vi "Solenoid GetSet.vi"(9 "Enum":enum16{"Set", "Get", "Clear"}(ring), 10 "PneumaticsDevRef in":T1={"Pneumatic State Reference"=refnum, "SolenoidDevRef"={"DevStatus"={"status"=FALSE, "code"=0, "source"=""}, "Pneumatics Control Module"=0, "Forward Solenoid Channel"=enum."Invalid", "Reverse Solenoid Channel"=enum."Invalid"}, "Pneumatic Configuration reference"=refnum}, 11 "DevRef":string) -> (0 "Error Out":errorcluster, 3 "PneumaticsDevRef out":T1={"Pneumatic State Reference"=refnum, "SolenoidDevRef"={"DevStatus"={"status"=FALSE, "code"=0, "source"=""}, "Pneumatics Control Module"=0, "Forward Solenoid Channel"=enum."Invalid", "Reverse Solenoid Channel"=enum."Invalid"}, "Pneumatic Configuration reference"=refnum})   [LabVIEW 2015]
uses:
  <userlib>/836-Library/Pneumatics/Pneumatics/836_PneumaticsDevRef.ctl
  <userlib>/836-Library/Pneumatics/Pneumatics/Pneumatic State.ctl
  <userlib>/836-Library/Pneumatics/Pneumatics/StateMachine.ctl
  <vilib>/Rock Robotics/WPI/Solenoid/WPI_SolenoidDevRef.ctl
  <vilib>/Rock Robotics/WPI/Solenoid/WPI_SolenoidChannel.ctl
  <userlib>/836-Library/Pneumatics/Pneumatics/Pneumatic Configuration.ctl
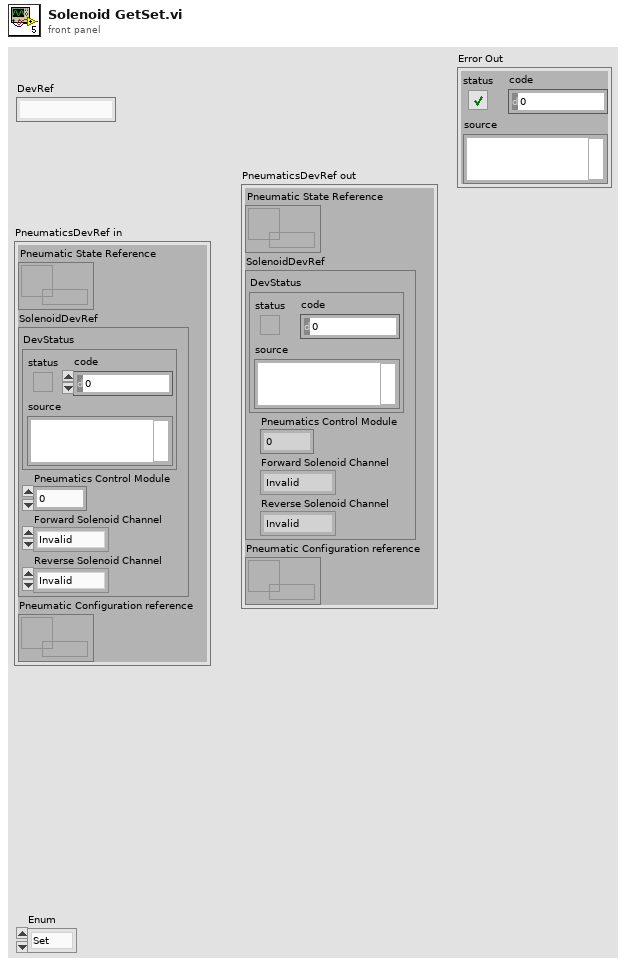
[diagram p1: front panel]
types:
  T1 = typedef "836_PneumaticsDevRef.ctl" = cluster{"Pneumatic State Reference":refnum<data-value>, "SolenoidDevRef":T2, "Pneumatic Configuration reference":refnum<data-value>}
  T2 = typedef "WPI_SolenoidDevRef.ctl" = cluster{"DevStatus":errorcluster, "Pneumatics Control Module":u8, "Forward Solenoid Channel":T3, "Reverse Solenoid Channel":T3}
  T3 = typedef "WPI_SolenoidChannel.ctl" = enum8{"Solenoid 0", "Solenoid 1", "Solenoid 2", "Solenoid 3", "Solenoid 4", "Solenoid 5", "Solenoid 6", "Solenoid 7", "Invalid"}
  T4 = typedef "Pneumatic State.ctl" = cluster{"Position":bool, "Initialize":bool, "Current State":T5, "Multiuse Timer A":u32, "Multiuse Timer B":u32}
  T5 = typedef "StateMachine.ctl" = enum8{"Status", "Forward", "Back", "Toggle", "Timed Forward", "Timed Back", "Analog Forwad", "Analog Back", "Digital Forward", "Digital Back", "Off", "Float", "Digital Forward Timeout", "Digital Back Timeout"}
  T6 = typedef "Pneumatic Configuration.ctl" = cluster{"Time Forward (ms)":u32, "Time Back (ms)":u32, "Digital Forward Time (ms)":u32, "Digital Backward Time (ms)":u32, "Analog Forward Settling Time (ms)":u32, "Analog Backward Settling Time (ms)":u32, "Analog Forward Threshold":sgl, "Analog Backward Threshold":sgl}
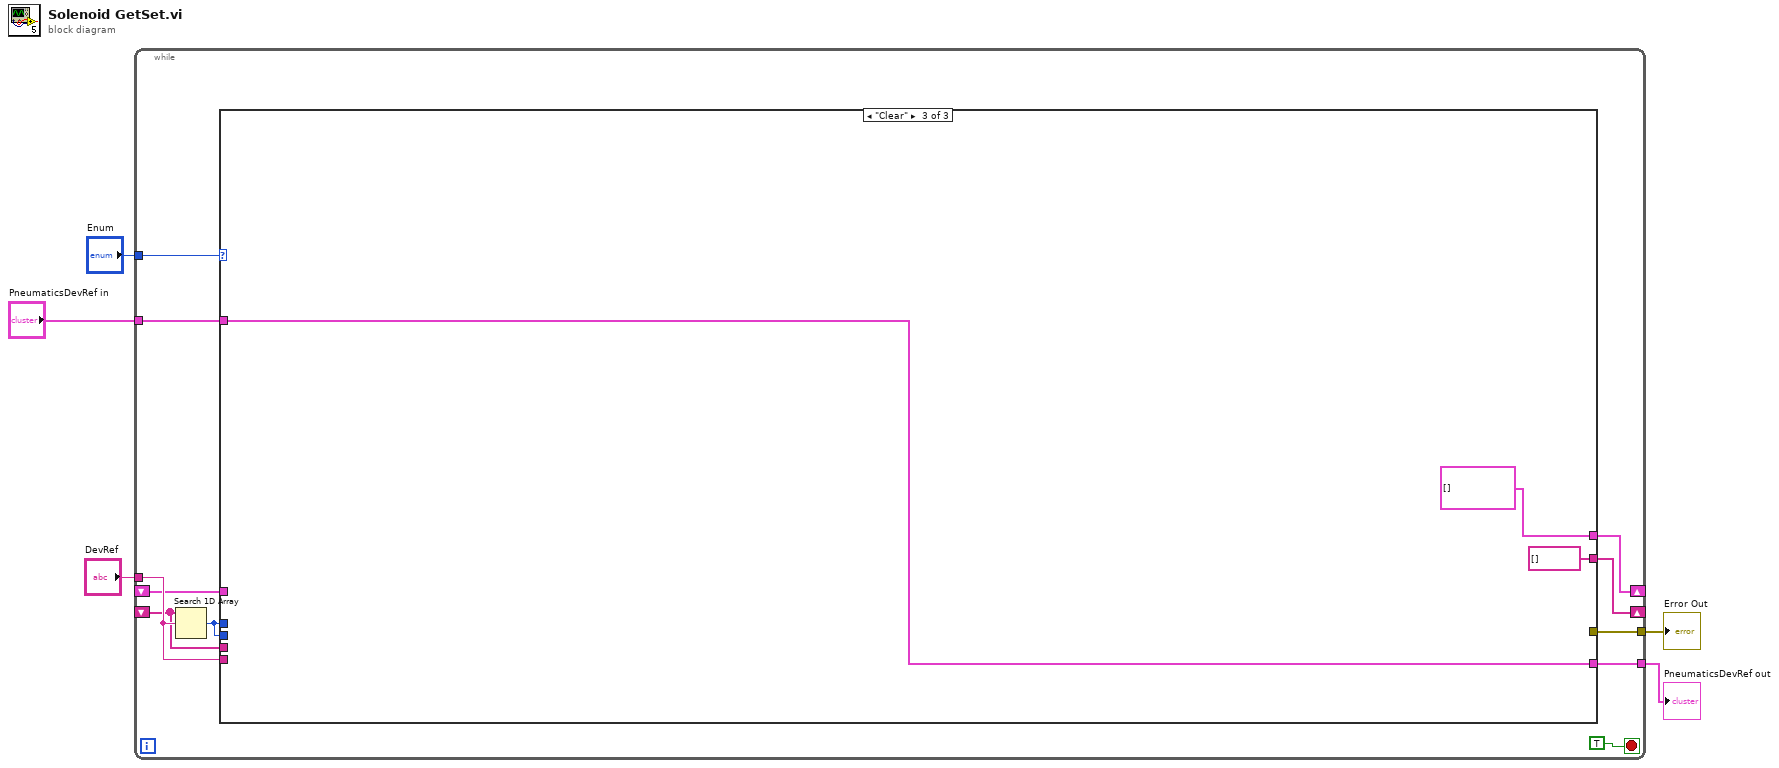
[diagram p0: block diagram]
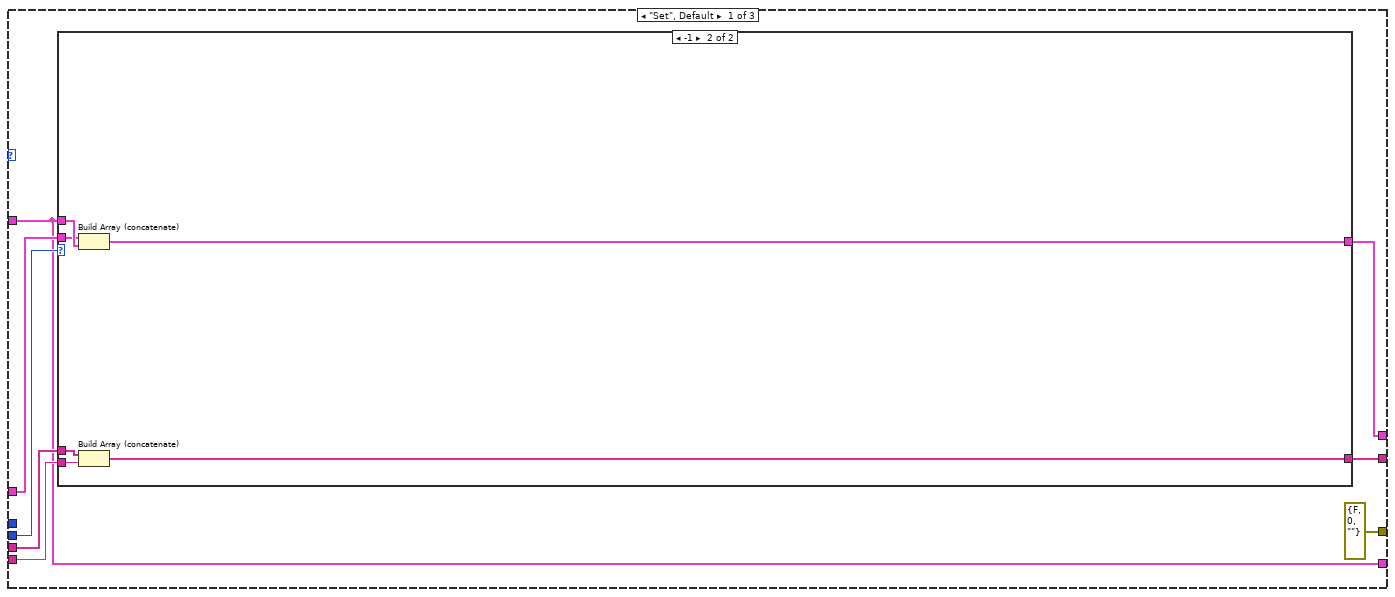
[diagram p2: hidden frame]
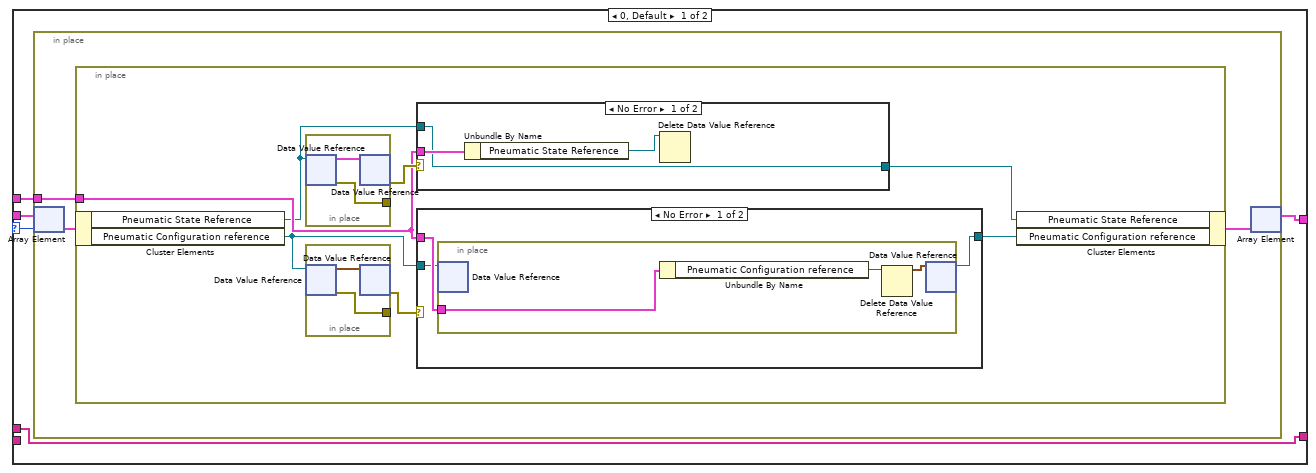
[diagram p3: hidden frame]
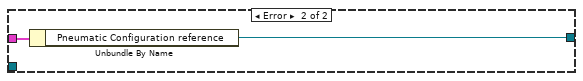
[diagram p4: hidden frame]
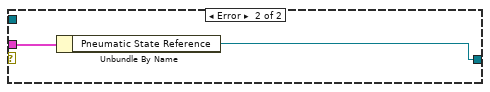
[diagram p5: hidden frame]
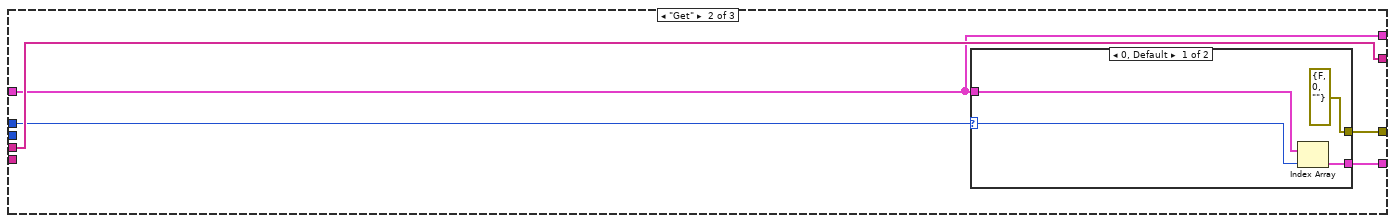
[diagram p6: hidden frame]
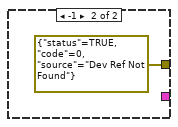
[diagram p7: hidden frame]
diagram:
  n1 = while {
    shift-right: [w12] -> _
    shift-left: _ -> [w11]
    shift-right: [w15] -> _
    shift-left: _ -> [w14]
    tunnel: "DevRef" -> [w16]
    tunnel: "PneumaticsDevRef in" -> [w13]
    tunnel: [w8] -> w4
    tunnel: "Enum" -> [w7]
    tunnel: [w6] -> w1
    stop <- TRUE stop-if-true
    n2 = Search 1D Array(1D array=w14, element=w16) -> (index of element=w9:i32)  [unwired: 1 out]
    n3 = case shown="\"Clear\"" w7 {
      tunnel: w9 -> [w24 _ _]
      tunnel: w16 -> [w23 _ _]
      tunnel: [w22 w67 string[] []] -> w15
      tunnel: w14 -> [w21 w67 _]
      tunnel: w13 -> [w18 _ w73]
      tunnel: [w20 w66 T1[] []] -> w12
      tunnel: w11 -> [w19 w66 _]
      tunnel: w9 -> [_ w65 _]
      tunnel: [w18 w64 w73] -> w8
      tunnel: [errorcluster {"status"=FALSE, "code"=0, "source"=""} ("error constant") w63 _] -> w6
      frame "Set", Default {
        n4 = case shown="-1" w24 {
          selector: w24 -> [w29 _]
          tunnel: [w25 w62] -> w20
          tunnel: [w28 w61] -> w22
          tunnel: w23 -> [_ w60]
          tunnel: w21 -> [w28 w59]
          tunnel: w18 -> [w26 w58]
          tunnel: w19 -> [w27 w57]
          frame 0, Default {
            n5 = in-place {
              in-place-border: w26 -> [w31]
              n6 = in-place-array #1(w27, w29) -> (w32:T1)
              n7 = in-place {
                in-place-border: w31 -> [w38]
                n8 = in-place-cluster #2(w32) -> ("Pneumatic State Reference"=w36:refnum<data-value>, "Pneumatic Configuration reference"=w35:refnum<data-value>)
                n9 = in-place {
                  in-place-border: [w56] -> _
                  n10 = in-place-dvr #3(w36) -> (w55:T4, w56:errorcluster)
                  n11 = in-place-dvr #3(w55) -> (w39:errorcluster)  [unwired: 1 out]
                }
                n12 = in-place {
                  in-place-border: [w54] -> _
                  n13 = in-place-dvr #4(w35) -> (w53:T6, w54:errorcluster)
                  n14 = in-place-dvr #4(w53) -> (w33:errorcluster)  [unwired: 1 out]
                }
                n15 = case shown="No Error" w39 {
                  tunnel: w38 -> [w50 w52]
                  tunnel: [w48 w51] -> w37
                  tunnel: w36 -> [w48 _]
                  frame No Error {
                    n16 = Unbundle By Name(w50) -> ("Pneumatic State Reference"=w49:refnum<data-value>)
                    n17 = Delete Data Value Reference(data value reference=w49) -> ()  [unwired: 1 in, 2 out]
                  }
                  frame Error {
                    n18 = Unbundle By Name(w52) -> ("Pneumatic State Reference"=w51:refnum<data-value>)
                  }
                }
                n19 = case shown="No Error" w33 {
                  tunnel: w38 -> [w42 w47]
                  tunnel: w35 -> [w41 _]
                  tunnel: [w40 w46] -> w34
                  frame No Error {
                    n20 = in-place {
                      in-place-border: w42 -> [w45]
                      n21 = in-place-dvr #5(w41) -> ()  [unwired: 2 out]
                      n22 = Unbundle By Name(w45) -> ("Pneumatic Configuration reference"=w44:refnum<data-value>)
                      n23 = Delete Data Value Reference(data value reference=w44) -> (data value=w43:T6)  [unwired: 1 in, 1 out]
                      n24 = in-place-dvr #5(w43) -> (w40:refnum<data-value>)  [unwired: 1 out]
                    }
                  }
                  frame Error {
                    n25 = Unbundle By Name(w47) -> ("Pneumatic Configuration reference"=w46:refnum<data-value>)
                  }
                }
                n26 = in-place-cluster #2("Pneumatic State Reference"=w37, "Pneumatic Configuration reference"=w34) -> (w30:T1)
              }
              n27 = in-place-array #1(w30) -> (w25:T1[])  [unwired: 1 out]
            }
          }
          frame -1 {
            n28 = Build Array (concatenate)(w57, w58) -> (w62:T1[])
            n29 = Build Array (concatenate)(w59, w60) -> (w61:string[])
          }
        }
      }
      frame "Get" {
        n30 = case shown="0, Default" w65 {
          selector: w65 -> [w70 _]
          tunnel: w66 -> [w71 _]
          tunnel: [w69 _] -> w64
          tunnel: [errorcluster {"status"=FALSE, "code"=0, "source"=""} ("error constant") errorcluster {"status"=TRUE, "code"=0, "source"="Dev Ref Not Found"} ("error constant")] -> w63
          frame 0, Default {
            n31 = Index Array(array=w71, index=w70) -> (element=w69:T1)
          }
          frame -1 {
          }
        }
      }
      frame "Clear" {
      }
    }
  }
  "PneumaticsDevRef out" <- w4
  "Error Out" <- w1
